vi "prefiltro.vi"(8 "pk-2":dbl, 9 "pk-1":dbl, 10 "rk-2":dbl) -> (2 "pk":dbl)   [LabVIEW 2019]
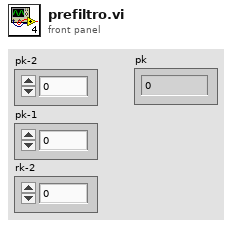
[diagram p1: front panel]
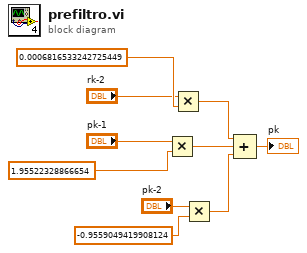
[diagram p0: block diagram]
diagram:
  n1 = Multiply(x="pk-1", y=1.95522328866654) -> (x*y=w8:dbl)
  n2 = Multiply(x="rk-2", y=0.0006816533242725449) -> (x*y=w9:dbl)
  n3 = Multiply(x="pk-2", y=-0.9559049419908124) -> (x*y=w7:dbl)
  n4 = Compound Arithmetic op=ADD(w9, w8, w7) -> (→"pk":dbl)
